vi "Convert Boolean to OnOff.vi"(10 "On/Off":bool, 11 "Initial String (\"\")":string) -> (3 "Resulting String":string)   [LabVIEW 2020, in "Yokogawa GX Series.lvlib"]
doc: "Converts boolean to \"On\" or \"Off\" and concatenate to string."
uses:
  <instrlib>/Yokogawa GX Series/Yokogawa GX Series.lvlib
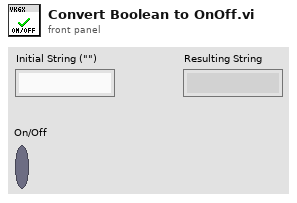
[diagram p1: front panel]
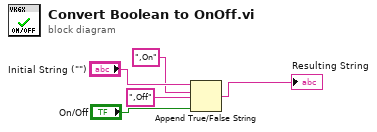
[diagram p0: block diagram]
diagram:
  n1 = Append True/False String(1:"On/Off", 2:",Off", 3:",On", 4:"Initial String (\"\")") -> (0:→"Resulting String":string)
